vi "Write_serial_log.vi"(1 "Log Type":string="SerLog_", 2 "Log Array":string[](array[string]), 3 "Header message":string, 4 "Channel Name":string) -> ()   [LabVIEW 2016]
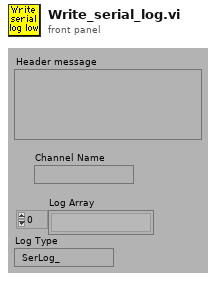
[diagram p1: front panel]
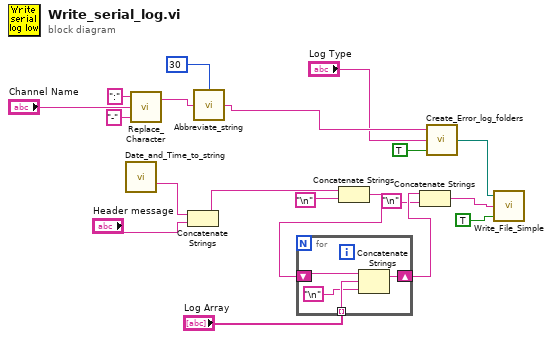
[diagram p0: block diagram]
diagram:
  n1 = call "Date_and_Time_to_string.vi"() -> ("Date and time (spreadsheet)"=w18:string)
  n2 = call "Replace_Character.vi"("Replace with"="-", "Input String"="Channel Name", "Search For"=":") -> ("Output string"=w7:string)  [unwired: 1 out]
  n3 = Concatenate Strings(w18, "Header message") -> (w17:string)
  n4 = call "Abbreviate_string.vi"("Input String"=w7, "Max String Length"=30) -> ("Output String"=w6:string)
  n5 = Concatenate Strings(w17, "\n") -> (w15:string)
  n6 = for {
    shift-right: [w22] -> w14
    shift-left: w15 -> [w23]
    tunnel: "Log Array" -> [w21] mode=indexing
    n7 = Concatenate Strings(w23, w21, "\n") -> (w22:string)
  }
  n8 = Concatenate Strings(w14, "\n") -> (w3:string)
  n9 = call "Create_Error_log_folders.vi"("Per Day Log File?"=TRUE, "Log Folder"="Log Type", "Log Filename"=w6) -> ("Server copy Location"=w1:path)  [unwired: 2 out]
  n10 = call "Write_File_Simple.vi"("append to file? (new file:F)"=TRUE, "character string"=w3, "file path"=w1) -> ()  [unwired: 2 out]
